vi "Read Language.vi"(8 "error in (no error)":errorcluster, 11 "Errors in":refnum<class "Errors.lvclass">) -> (0 "error out":errorcluster, 2 "Language":T1, 3 "Errors out":refnum<class "Errors.lvclass">)   [LabVIEW 2013, in "Error-handling.lvlib" / "Errors.lvclass"]
uses:
  Errors.lvclass
  Languages.ctl
  Errors.lvclass/Errors.ctl
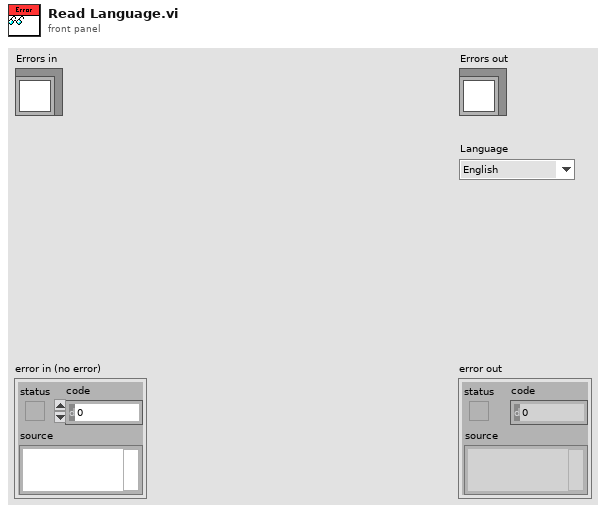
[diagram p1: front panel]
types:
  T1 = typedef "Error-handling.lvlib/Errors.lvclass/Languages.ctl" = enum16{"English"}
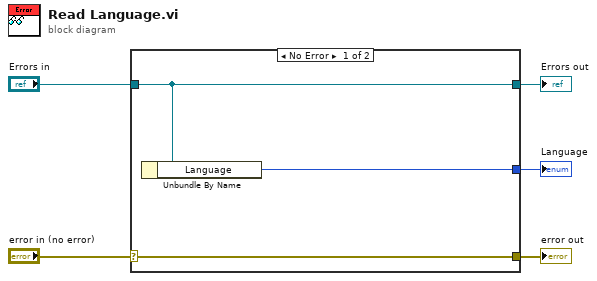
[diagram p0: block diagram]
diagram:
  n1 = case shown="No Error" "error in (no error)" {
    selector: "error in (no error)" -> [w8 w9]
    tunnel: [w8 w9] -> w4
    tunnel: [w7 w10] -> w2
    tunnel: "Errors in" -> [w7 w10]
    tunnel: [w6 _] -> w1
    frame No Error {
      n2 = Unbundle By Name(w7) -> ("Language"=w6:T1)
    }
    frame Error {
    }
  }
  "error out" <- w4
  "Errors out" <- w2
  "Language" <- w1
